vi "Reload.vi"(0 "reference in":refnum<class "DP_WebView.lvclass">, 5 "Error In":errorcluster) -> (14 "reference out":refnum<class "DP_WebView.lvclass">, 19 "Error Out":errorcluster)   [LabVIEW 2020, in "DP_WebView.lvclass"]
uses:
  DP_WebView.lvclass
  C:/Projects/DependencyViewer/DependencyViewer/DP_WebView_class/data/Microsoft.Web.WebView2.Core.dll
  data/Microsoft.Web.WebView2.Core.dll
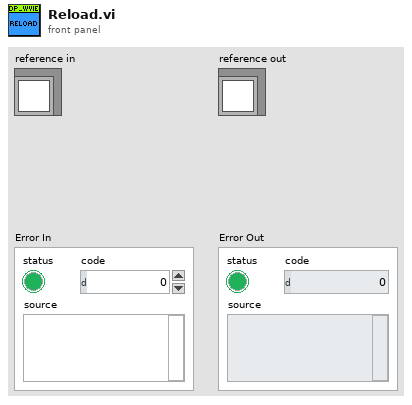
[diagram p1: front panel]
types:
  T1 = typedef "DP_WebView.lvclass/ObjectAttributes.ctl" = cluster{"WebView Container":refnum<k24>, "CoreWebViewRef":refnum<k24>, "Status":i32, "Status Message":string, "User Data Folder":path, "BrowserProcessId":u32}
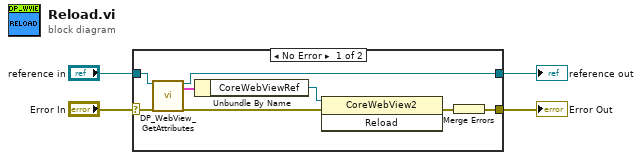
[diagram p0: block diagram]
diagram:
  n1 = case shown="No Error" "Error In" {
    selector: "Error In" -> [w12 w14]
    tunnel: [w9 w14] -> w3
    tunnel: [w10 w13] -> w1
    tunnel: "reference in" -> [w11 w13]
    frame No Error {
      n2 = call "DP_WebView_GetAttributes.vi"("reference in"=w11, "error in (no error)"=w12) -> ("reference out"=w10:refnum<class "DP_WebView.lvclass">, "Data"=w8:T1, "error out"=w6:errorcluster)  [unwired: 14 in, 1 out]
      n3 = Unbundle By Name(w8) -> ("CoreWebViewRef"=w7:refnum<k24>)
      n4 = invoke class="CoreWebView2" method="Reload"(reference=w7, error in=w6) -> (error out=w5:errorcluster)  [unwired: 1 in, 2 out]
      n5 = Merge Errors(w5) -> (w9:errorcluster)
    }
    frame Error {
    }
  }
  "Error Out" <- w3
  "reference out" <- w1
